vi "CreateEvent.vi"(11 "eventDescription":string) -> (3 "EventData":refnum<class "EventData.lvclass">)   [LabVIEW 2016, in "Event Logging.lvlib" / "EventData.lvclass"]
uses:
  EventData.lvclass
  Types/EventType.ctl
  EventData.lvclass/EventData.ctl
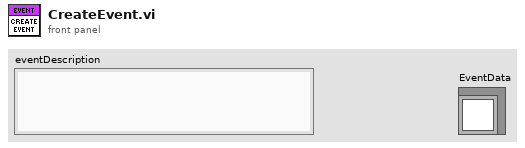
[diagram p1: front panel]
types:
  T1 = typedef "Event Logging.lvlib/EventData.lvclass/EventType.ctl" = enum16{"Event", "Warning", "Error"}
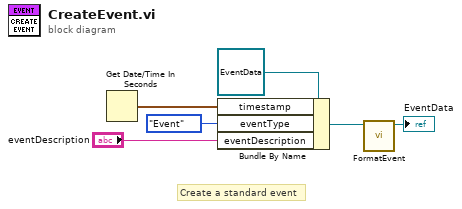
[diagram p0: block diagram]
diagram:
  # "Create a standard event"
  n1 = Get Date/Time In Seconds() -> (seconds since 1Jan1904=w5:timestamp)
  n2 = Bundle By Name(cluster=refnum<class "EventData.lvclass"> refnum ("Event Logging.lvlib:EventData.lvclass"), "timestamp"=w5, "eventType"=EventType."Event", "eventDescription"="eventDescription") -> (w2:refnum<class "EventData.lvclass">)
  n3 = call-dynamic "FormatEvent.vi"("EventData in"=w2) -> ("EventData out"=→"EventData":refnum<class "EventData.lvclass">)  [unwired: 10 in]
